vi "InitMultipleDevices.vi"(4 "error in (no error)":errorcluster, 6 "msecDelayForDiscovery":i32=800) -> (0 "error out":errorcluster, 3 "CmdLib Out":refnum<k24>)   [LabVIEW 2020]
uses:
  C:/GEECS/Developers Version/builds/Device builds/Picomotor8742dotNet/CmdLib.dll
  CmdLib.dll
panel:
  out "deviceKeys":string[](array[string])
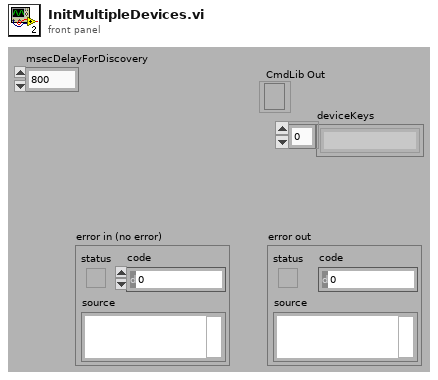
[diagram p1: front panel]
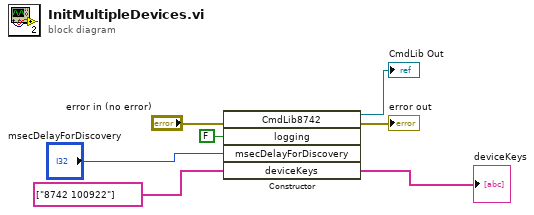
[diagram p0: block diagram]
diagram:
  n1 = constructor class="CmdLib8742"(error in="error in (no error)", "logging"=FALSE, "msecDelayForDiscovery"="msecDelayForDiscovery", "deviceKeys"=string[] ["8742 100922"]) -> (reference out=→"CmdLib Out":refnum<k24>, error out=→"error out":errorcluster, "deviceKeys"=→"deviceKeys":string[])  [unwired: 2 in, 3 out]
